vi "Send Messages.vi"(6 "Reply to...":refnum<class "Send.lvclass">, 8 "error in (no error)":errorcluster, 10 "Messages":refnum<class "MSG.lvclass">[](array[class]), 11 "MSR Parent in":refnum<class "Send.lvclass">) -> (0 "error out":errorcluster, 3 "MSR Parent out":refnum<class "Send.lvclass">)   [LabVIEW 2011, in "Messenging.lvlib" / "Send.lvclass"]
uses:
  Send.lvclass
  TextVarientMessage/MSG.lvclass
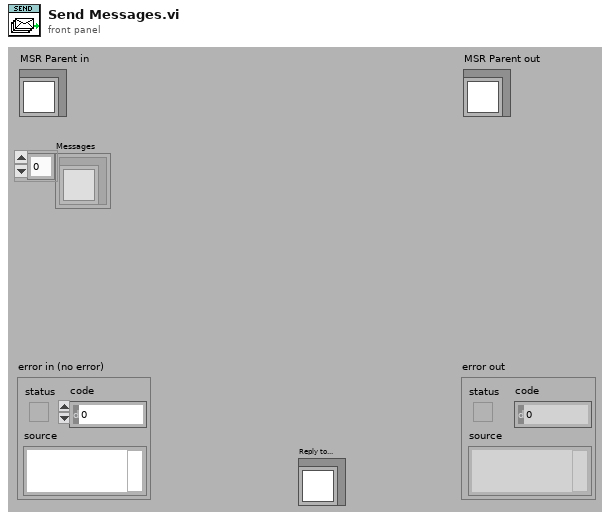
[diagram p1: front panel]
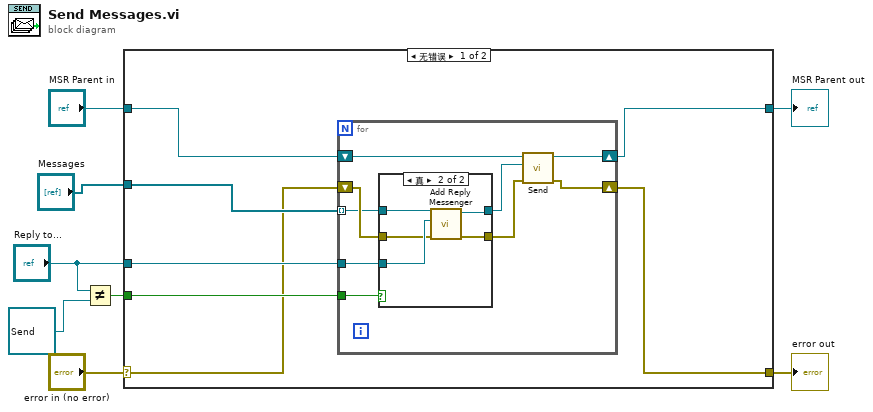
[diagram p0: block diagram]
diagram:
  n1 = Not Equal?(x="Reply to...", y=refnum<class "Send.lvclass"> refnum) -> (x != y?=w2:bool)
  n2 = case shown="无错误" "error in (no error)" {
    selector: "error in (no error)" -> [w9 w33]
    tunnel: [w13 w33] -> w7
    tunnel: [w14 w32] -> w5
    tunnel: "MSR Parent in" -> [w15 w32]
    tunnel: "Messages" -> [w10 _]
    tunnel: w2 -> [w12 _]
    tunnel: "Reply to..." -> [w11 _]
    frame No Error {
      n3 = for {
        shift-right: [w23] -> w14
        shift-left: w15 -> [w24]
        shift-right: [w22] -> w13
        shift-left: w9 -> [w21]
        tunnel: w12 -> [w16]
        tunnel: w11 -> [w17]
        tunnel: w10 -> [w19] mode=indexing
        n4 = case shown="真" w16 {
          tunnel: w19 -> [w25 w31]
          tunnel: w17 -> [_ w30]
          tunnel: w21 -> [w26 w29]
          tunnel: [w26 w28] -> w20
          tunnel: [w25 w27] -> w18
          frame False {
          }
          frame True {
            n5 = call "Add Reply Messenger.vi"("error in (no error)"=w29, "Reply to..."=w30, "Message"=w31) -> ("error out"=w28:errorcluster, "Message"=w27:refnum<class "MSG.lvclass">)  [unwired: 7 out]
          }
        }
        n6 = call-dynamic "Send.vi"("error in (no error)"=w20, "Message"=w18, "MSR Parent in"=w24) -> ("error out"=w22:errorcluster, "MSR Parent out"=w23:refnum<class "Send.lvclass">)  [unwired: 7 out]
      }
    }
    frame Error {
    }
  }
  "error out" <- w7
  "MSR Parent out" <- w5
